vi "formatstr.vi"(1 "command in":string) -> (0 "Formated command string":string)   [LabVIEW 2017]
doc: "Formats the command into a string acceptable to the instrument"
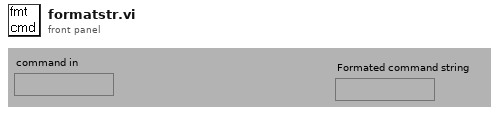
[diagram p1: front panel]
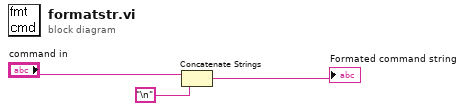
[diagram p0: block diagram]
diagram:
  n1 = Concatenate Strings("command in", "\n") -> (→"Formated command string":string)
